vi "setup_for_rot.vi"(7 "RON settings":T1={"RON Affected axes"=[], "Reference mode"=[], "Check FRF?"=TRUE}, 8 "错误输入（无错误）":errorcluster, 9 "USB settings for rotation":cluster{"S/N":string, "USB Search?":bool}={"S/N"="0135500392", "USB Search?"=FALSE}, 10 "DaisyChain settings for rotation":T2={"Register DC"=FALSE, "DaisyChain Search?"=TRUE, "Device ID"=1}, 11 "System no.输入":i32=1 min=1 step=1) -> (0 "错误输出":errorcluster, 2 "Conn. \nAxes":string[](array[string]), 3 "System no. 3":i32)   [LabVIEW 2017]
panel:
  out "Position":dbl[](array[numeric]) format="%.6f"
  out "Device ID out":i32
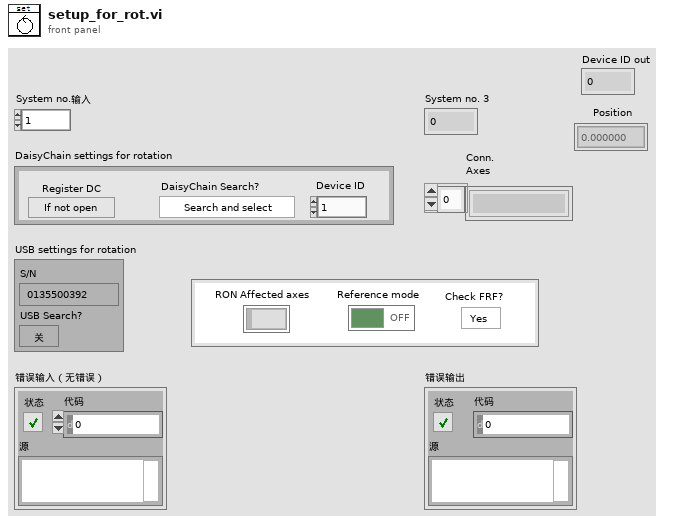
[diagram p1: front panel]
types:
  T1 = cluster{"RON Affected axes":string[], "Reference mode":bool[], "Check FRF?":bool}
  T2 = cluster{"Register DC":bool, "DaisyChain Search?":bool, "Device ID":i32}
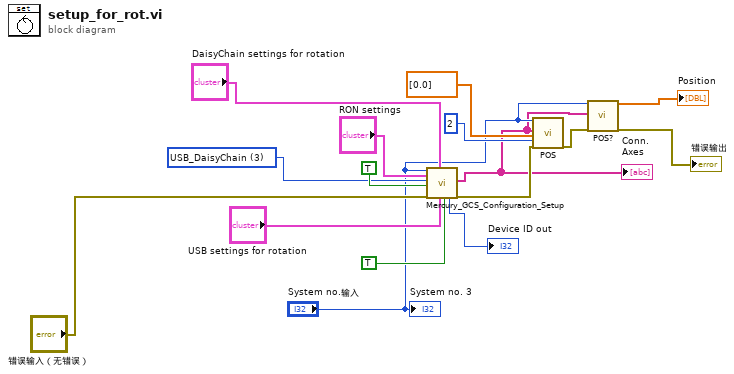
[diagram p0: block diagram]
diagram:
  w12 = u16 3 items=["RS232", "RS232 DaisyChain", "USB", "USB_DaisyChain"] ("Interface")
  n1 = call "Mercury_GCS_Configuration_Setup.vi"("System no."="System no.输入", "RON settings"="RON settings", "Interface"=w12, "All axes?"=TRUE ("Switch servo on?"), "error in"="错误输入（无错误）", "DaisyChain settings"="DaisyChain settings for rotation", "USB settings"="USB settings for rotation", "Switch servo on?"=TRUE) -> ("Device ID out"=→"Device ID out":i32, "Conn. \nAxes"=w3:string[], "error out"=w8:errorcluster)  [unwired: 5 in, 4 out]
  "Conn. \nAxes" <- w3
  n2 = call "POS.vi"("System no."="System no.输入", "Axes to set"=w3, "Position values"=dbl[] [0.0], "No.of digits"=i16 2, "error in"=w8) -> ("error out"=w5:errorcluster)  [unwired: 14 in]
  n3 = call "POS?.vi"("System no."="System no.输入", "Axes to query"=w3, "error in"=w5) -> ("Position"=→"Position":dbl[], "error out"=→"错误输出":errorcluster)  [unwired: 15 in]
  "System no. 3" <- "System no.输入"
